vi "m1m3_logEvent_AppliedCylinderForces.vi"(8 "error in (no error)":errorcluster, 11 "logevent_AppliedCylinderForces_Ctl":T1) -> (0 "error out":errorcluster, 2 "function return":i32, 3 "logevent_AppliedCylinderForces_Ctl out":T1)   [LabVIEW 2016, in "SALLV_m1m3.lvlib"]
doc: "int m1m3_shm_logEvent_AppliedCylinderForcesLV(m1m3_logevent_AppliedCylinderForcesLV *logevent_AppliedCylinderForces_Ctl );"
uses:
  SALLV_m1m3.lvlib
  DataTypes/logevent_AppliedCylinderForces.ctl
  SALLV_m1m3.so
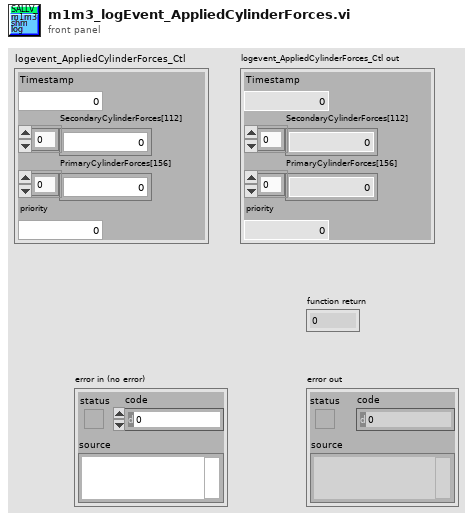
[diagram p1: front panel]
types:
  T1 = typedef "SALLV_m1m3.lvlib/logevent_AppliedCylinderForces.ctl" = cluster{"Timestamp":dbl, "SecondaryCylinderForces[112]":i32[], "PrimaryCylinderForces[156]":i32[], "priority":i32}
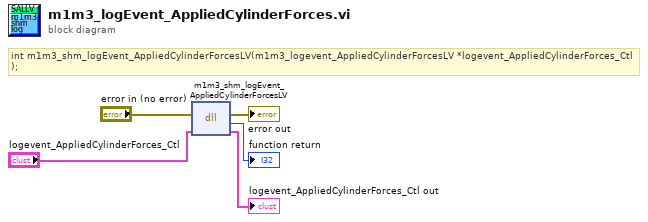
[diagram p0: block diagram]
diagram:
  # "int m1m3_shm_logEvent_AppliedCylinderForcesLV(m1m3_logevent_AppliedCylinderForcesLV *logevent_AppliedCylinderForces_Ctl );"
  n1 = dll-call lib="opt/CODE/SALLV_m1m3/SALLV_m1m3.*" fn="m1m3_shm_logEvent_AppliedCylinderForcesLV"(error in="error in (no error)", "logevent_AppliedCylinderForces_Ctl"="logevent_AppliedCylinderForces_Ctl") -> (error out=→"error out":errorcluster, →"function return":i32, "logevent_AppliedCylinderForces_Ctl"=→"logevent_AppliedCylinderForces_Ctl out":T1)  [unwired: 2 in, 1 out]
